vi "ZT.vi"(6 "Numeric":dbl, 7 "Thermal Conductivity":dbl, 9 "Seebeck Coe":dbl, 10 "Numeric 2":dbl, 11 "Numeric 3":dbl) -> (3 "ZT":dbl)   [LabVIEW 2020]
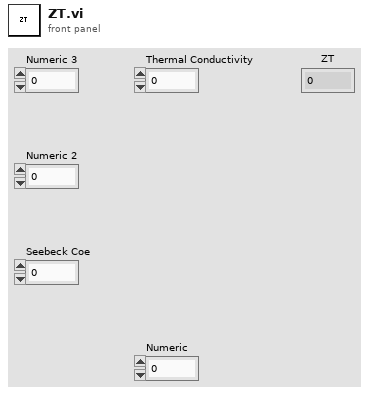
[diagram p1: front panel]
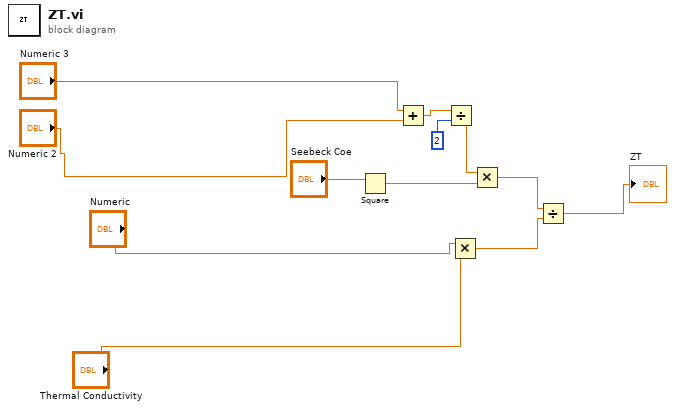
[diagram p0: block diagram]
diagram:
  n1 = Square(x="Seebeck Coe") -> (x^2=w7:dbl)
  n2 = Add(x="Numeric 3", y="Numeric 2") -> (x+y=w4:dbl)
  n3 = Divide(x=w4, y=2) -> (x/y=w6:dbl)
  n4 = Multiply(x="Numeric", y="Thermal Conductivity") -> (x*y=w11:dbl)
  n5 = Multiply(x=w6, y=w7) -> (x*y=w10:dbl)
  n6 = Divide(x=w10, y=w11) -> (x/y=→"ZT":dbl)
